vi "Read all vectors.vi"(8 "error in (no error)":errorcluster, 11 "AER in":refnum<class "AER.lvclass">) -> (0 "error out":errorcluster, 1 "Pre IDs":i32[](array[numeric]), 2 "No Pre":i32[](array[numeric]), 3 "AER out":refnum<class "AER.lvclass">, 4 "W":dbl[](array[numeric]), 5 "Currents":dbl[](array[numeric]), 6 "No N":i32[](array[numeric]))   [LabVIEW 2013, in "AER.lvclass"]
uses:
  AER.lvclass
  AER.lvclass/AER.ctl
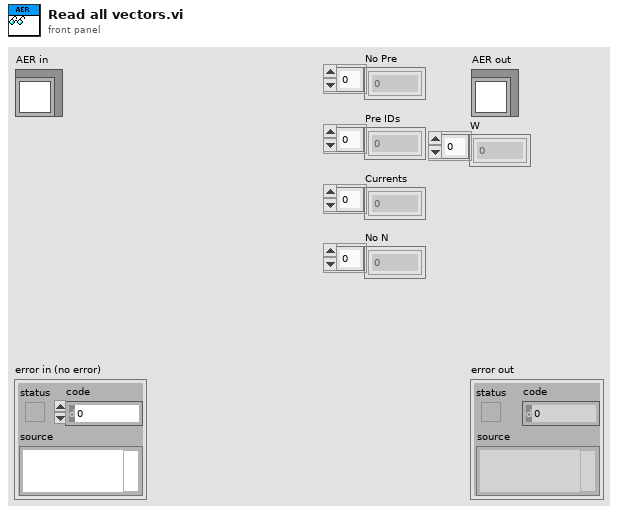
[diagram p1: front panel]
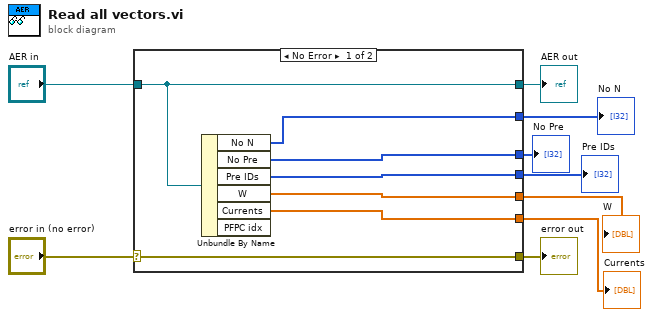
[diagram p0: block diagram]
diagram:
  n1 = case shown="No Error" "error in (no error)" {
    selector: "error in (no error)" -> [w16 w17]
    tunnel: [w16 w17] -> w8
    tunnel: [w15 w18] -> w6
    tunnel: "AER in" -> [w15 w18]
    tunnel: [w14 _] -> w5
    tunnel: [w13 _] -> w4
    tunnel: [w12 _] -> w3
    tunnel: [w11 _] -> w2
    tunnel: [w10 _] -> w1
    frame No Error {
      n2 = Unbundle By Name(w15) -> ("No N"=w10:i32[], "No Pre"=w14:i32[], "Pre IDs"=w13:i32[], "W"=w12:dbl[], "Currents"=w11:dbl[])  [unwired: 1 out]
    }
    frame Error {
    }
  }
  "error out" <- w8
  "AER out" <- w6
  "No Pre" <- w5
  "Pre IDs" <- w4
  "W" <- w3
  "Currents" <- w2
  "No N" <- w1
